vi "locate control module.vi"(10 "name":string, 11 "user module configuration in":refnum<class "user tag bus module configuration.lvclass">) -> (0 "module duplicate":T1={"name"="", "setpoint"=refnum, "process variable"=refnum, "output"=refnum, "gains"={"Kp"=0.0, "Ki"=0.0, "Kd"=0.0}, "output range"={"output high"=100.0, "output low"=-100.0}} {"output range"."output low" format="%.2f"; "output range"."output high" format="%.2f"}, 1 "index":i32, 2 "found":bool, 3 "user module configuration out":refnum<class "user tag bus module configuration.lvclass">)   [LabVIEW 2013, in "user tag bus module configuration.lvclass"]
uses:
  user tag bus module configuration.lvclass
  control module configuration.ctl
  <vilib>/NI/Tag Bus Module Framework/channel/TBM channel.lvclass
  gains.ctl
  user tag bus module configuration.lvclass/user tag bus module configuration.ctl
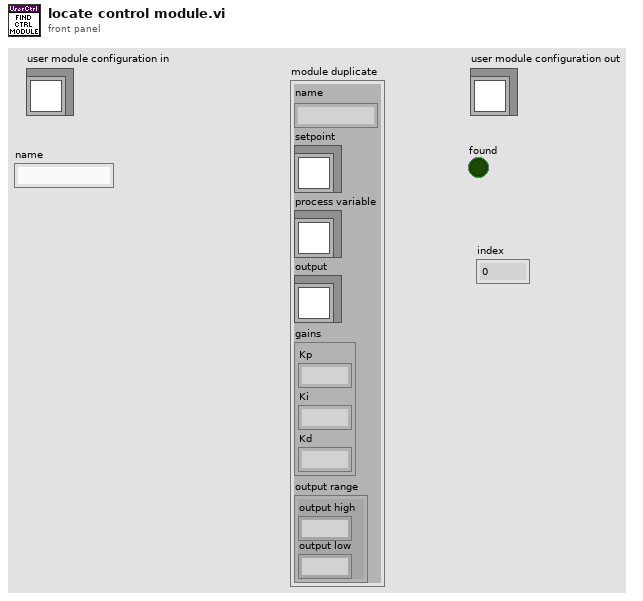
[diagram p1: front panel]
types:
  T1 = typedef "user tag bus module configuration.lvclass/control module configuration.ctl" = cluster{"name":string, "setpoint":refnum<class "TBM channel.lvclass">, "process variable":refnum<class "TBM channel.lvclass">, "output":refnum<class "TBM channel.lvclass">, "gains":T2, "output range":cluster{"output high":dbl, "output low":dbl}}
  T2 = typedef "user tag bus module configuration.lvclass/gains.ctl" = cluster{"Kp":dbl, "Ki":dbl, "Kd":dbl}
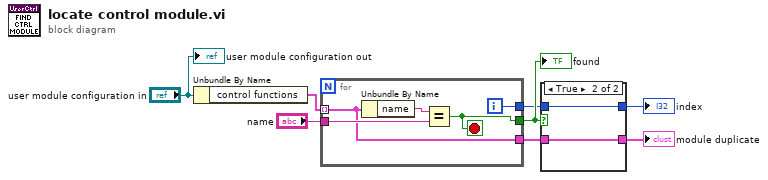
[diagram p0: block diagram]
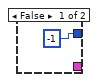
[diagram p2: hidden frame]
diagram:
  n1 = Unbundle By Name("user module configuration in") -> ("control functions"=w7:T1[])
  n2 = for {
    tunnel: w7 -> [w10] mode=indexing
    tunnel: "name" -> [w13]
    tunnel: [w11] -> w2
    tunnel: [w10] -> w4
    tunnel: [w9] -> w6
    i -> [w11]
    stop <- w9 stop-if-true
    n3 = Unbundle By Name(w10) -> ("name"=w12:string)
    n4 = Equal?(x=w12, y=w13) -> (x = y?=w9:bool)
  }
  "found" <- w6
  n5 = case shown="True" w6 {
    tunnel: [_ w16] -> w3
    tunnel: w4 -> [_ w16]
    tunnel: [-1 w15] -> w1
    tunnel: w2 -> [_ w15]
    frame False {
    }
    frame True {
    }
  }
  "module duplicate" <- w3
  "index" <- w1
  "user module configuration out" <- "user module configuration in"
